vi "Initial Values-Unbundler-Strings.vi"(8 "error in (no error)":errorcluster, 9 "Keys Array":T2, 10 "Section name":string, 11 "User profile ini file ref":T1) -> (0 "error out":errorcluster, 3 "User profile ini file ref":T1)   [LabVIEW 2017]
uses:
  <vilib>/Utility/config.llb/Config Data RefNum.ctl
  Typedefs/Ini file interface (String).ctl
  Global Variables/gl_UI Ctrl Refs.vi
  <vilib>/Utility/config.llb/NI_LVConfig.lvlib
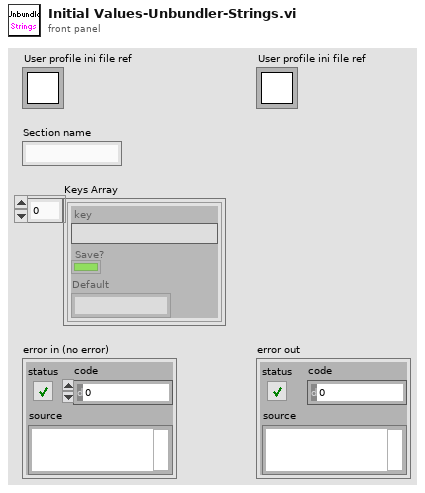
[diagram p1: front panel]
types:
  T1 = typedef "NI_LVConfig.lvlib/Config Data RefNum.ctl" = refnum<k1>
  T2 = typedef "Ini file interface (String).ctl" = cluster{"key":string, "Save?":bool, "Default":string}[]
  T3 = typedef "UI ctrl refs cluster.ctl" = cluster{"Top level VI path":path, "Top level VI ref":refnum<vi>, "User menu ref":refnum<k9>, "Sub Panel control":refnum<vi>, "Imaging Param Tab":refnum<vi>, "Occurrence-Start drivers":refnum<k4>, "Occurrence-Speed logging initialised":refnum<k4>, "Occurrence-XYZ stage initialised":refnum<k4>, "Exit button":refnum<vi>, "Status ind":refnum<vi>, "Set as origin":refnum<vi>, "Speed Logging":refnum<vi>, "Time Lapse":refnum<vi>, "Live Imaging":refnum<vi>, "AOL Z Stack":refnum<vi>, "Motor Z Stack":refnum<vi>, "Funct Acq button":refnum<vi>, "Hard Shutter":refnum<vi>, "Virtual Shutter":refnum<vi>, "Laser Power":refnum<vi>, "AOL Mode":refnum<vi>, "Frame Size":refnum<vi>, "Field of View":refnum<vi>, "Dwell Time":refnum<vi>, "Zoom":refnum<vi>, "AOL Z":refnum<vi>, "Objective":refnum<vi>, "Axis":refnum<vi>, "Paths & Names":refnum<vi>, "Experiment folder path (ind.)":refnum<vi>, "Last State (Ind.)":refnum<vi>, "Averages":refnum<vi>, "Angle (degrees)":refnum<vi>, "X centre":refnum<vi>, "Y centre":refnum<vi>, "Plane Mode":refnum<vi>, "# Planes":refnum<vi>, "Z Start":refnum<vi>, "Z Stop":refnum<vi>, "Z Step":refnum<vi>, "PMT 1":refnum<vi>, "PMT 2":refnum<vi>, "Stage XYZ Position":refnum<vi>, "Pockels@Z Start":refnum<vi>, "Pockels@Z Stop":refnum<vi>, "Obtain Z Start":refnum<vi>, "Obtain Z Stop":refnum<vi>, "Live stim.trig.period":refnum<vi>, "Live stim.trig.enable":refnum<vi>, "Movement Correction":refnum<vi>, "Load Reference Image":refnum<vi>, "XY Stage Move":refnum<vi>, "MovCor Cluster":refnum<vi>, "RefDAQParam":refnum<vi>, "Funct. Acq. Pockels Modulation":refnum<vi>, "Background MovCor":refnum<vi>, "Ref Laser Power":refnum<vi>, "Enable Video Recording":refnum<vi>, "Video Record-Live Imaging":refnum<vi>, "Video Record-Funct acq":refnum<vi>, "Reference Source":refnum<vi>, "AOL Z-stack Chirps Ready (ind)":refnum<vi>, "Target time between mov.cor. ref triggers (ms)":refnum<vi>, "Funct. Acq. Ref frame save":refnum<vi>, "Tracking button":refnum<vi>, "Show ref plots window":refnum<vi>, "Center freq ind (nm)":refnum<vi>, "Pickup mode (ind)":refnum<vi>, "Logging queue (ind)":refnum<vi>, "Back aperture power (ind.)":refnum<vi>, "Power after objective (ind.)":refnum<vi>, "Switch user":refnum<vi>, "Ls1 Conn. Status":refnum<vi>, "Ls1Tuning Status":refnum<vi>, "Ls1 Faults":refnum<vi>, "Ls1 Connection":refnum<vi>, "Ls1 Mode":refnum<vi>, "Ls1 POWER [mW]":refnum<vi>, "Ls1Shutter":refnum<vi>, "Ls1 Wavelength":refnum<vi>, "Ls1 Note":refnum<vi>, "Ls1 Confirm Wav":refnum<vi>, "Ls1 PreChrp Prism1":refnum<vi>, "Ls1 PreChrp Prism2":refnum<vi>, "Ls1 wav top Ind":refnum<vi>, "Ls1 power top Ind":refnum<vi>, "Ls1 Pump peak Hold":refnum<vi>, "Ls1 Status Ind":refnum<vi>, "Ls1 wav cancel":refnum<vi>, "Experiment Type":refnum<vi>, "Biology Information":refnum<vi>}
  T4 = cluster{"Base Directory":path, "User folder?":bool, "Sub-Folder":string, "Experiment folder custom name":string}
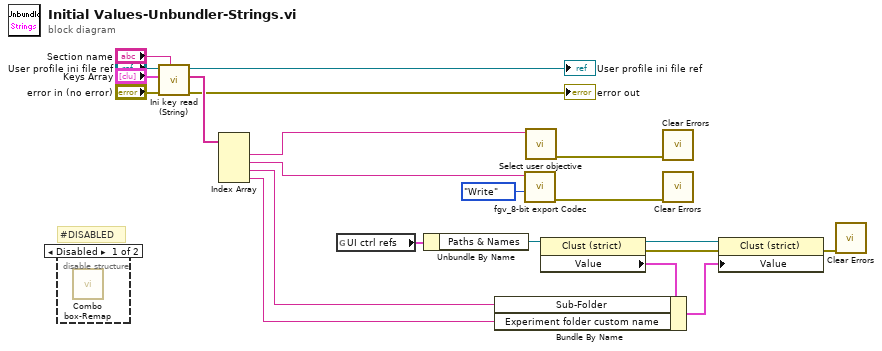
[diagram p0: block diagram]
diagram:
  # "#DISABLED"
  n1 = disable-structure shown="Disabled" {
    frame Disabled {
      n2 = call "Combo box-Remap.vi"() -> ()  [unwired: 11 in, 1 out]
    }
    frame Enabled {
    }
  }
  n3 = call "Ini key read (String).vi"("Section name"="Section name", "error in (no error)"="error in (no error)", "Keys setup"="Keys Array", "Ini file ref in"="User profile ini file ref") -> ("error out"=→"error out":errorcluster, "Value read/used"=w21:string[], "Ini file ref"=→"User profile ini file ref":T1)  [unwired: 5 in]
  n4 = Index Array(array=w21) -> (element #1=w1:string, element #2=w13:string, element #3=w5:string, element #4=w4:string)  [unwired: 4 in]
  n5 = global read "gl_UI Ctrl Refs.vi" "UI ctrl refs"() -> (w6:T3)
  n6 = Unbundle By Name(w6) -> ("Paths & Names"=w11:refnum<vi>)
  n7 = call "fgv_8-bit export Codec.vi"("Function"=enum16{"Intialize", "Write", "Read", "Clear"}."Write", "Codec"=w13) -> ("error out"=w12:errorcluster)  [unwired: 8 in, 1 out]
  n8 = call "Select user objective.vi"("User objective"=w1) -> ("error out"=w2:errorcluster)  [unwired: 10 in]
  n9 = property on="Property Node" class="Clust (strict)"(reference=w11) -> (reference out=w3:refnum<vi>, error out=w10:errorcluster, "Value"=w8:T4)  [unwired: 1 in]
  n10 = Bundle By Name(cluster=w8, "Sub-Folder"=w5, "Experiment folder custom name"=w4) -> (w7:T4)
  n11 = call <vilib>:"Clear Errors.vi"("error in (no error)"=w2) -> ()  [unwired: 5 in, 2 out]
  n12 = call <vilib>:"Clear Errors.vi"("error in (no error)"=w12) -> ()  [unwired: 5 in, 2 out]
  n13 = property on="Property Node" class="Clust (strict)"(reference=w3, error in=w10, "Value"=w7) -> (error out=w9:errorcluster)  [unwired: 1 out]
  n14 = call <vilib>:"Clear Errors.vi"("error in (no error)"=w9) -> ()  [unwired: 5 in, 2 out]
